vi "_DServerStart.vi"(3 "error in":errorcluster, 4 "instance name":string="unspecified_instance_name", 5 "executable name":string="unspecified_application_name") -> (0 "error out":errorcluster, 1 "device_list":string[](array[string]), 2 "dserver evt.":T1)   [LabVIEW 2014, in "tango.lvlib"]
uses:
  tango.lvlib
  Client Request Handling/Typedefs/_DServerEvent.ctl
  Client Request Handling/Typedefs/_DServerClientRequest.ctl
  Client Request Handling/Typedefs/_DServerClientRequestType.ctl
  Client Request Handling/Typedefs/_DServerClientRequestData.ctl
  Client Request Handling/Typedefs/_GenericDataBuffer.ctl
  Common VIs/Typedefs/_AttributeDataType_t.ctl
  tango_binding.so
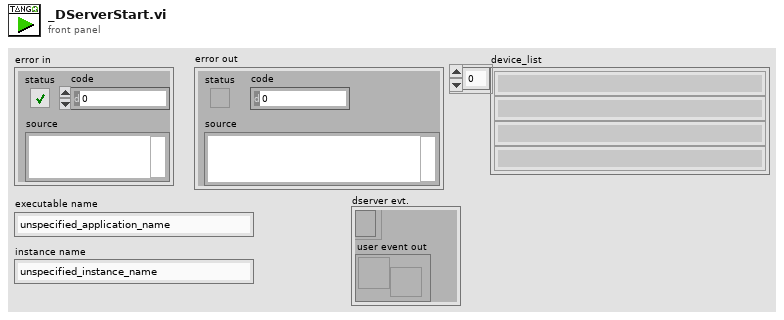
[diagram p1: front panel]
types:
  T1 = typedef "tango.lvlib/_DServerEvent.ctl" = cluster{"event registration refnum":refnum<event-registration>, "user event out":refnum<user-event>}
  T2 = cluster{"event registration refnum":refnum<event-registration>, "user event out":refnum<user-event>}
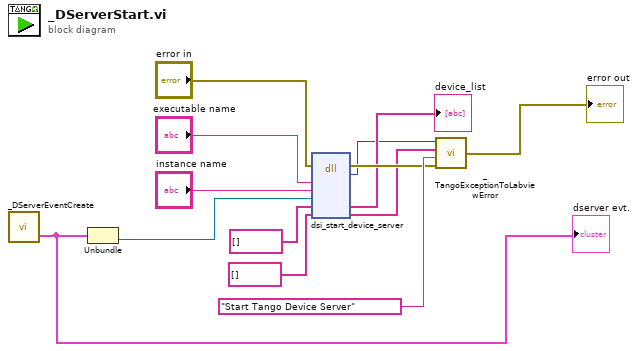
[diagram p0: block diagram]
diagram:
  n1 = call "_DServerEventCreate.vi"() -> ("dserver evt."=w1:T2)  [unwired: 1 in, 1 out]
  "dserver evt." <- w1
  n2 = Unbundle(w1) -> ("user event out"=w2:refnum<user-event>)  [unwired: 1 out]
  n3 = dll-call lib="tango_binding.*" fn="dsi_start_device_server"(error in="error in", "executable_name"="executable name", "instance_name"="instance name", "devicer_server_evt_ref"=w2, "device_list"=string[] [] ("error stack"), "error_stack"=string[] [] ("error stack")) -> (error out=w11:errorcluster, "return type"=w5:i32, "device_list"=→"device_list":string[], "error_stack"=w4:string[])  [unwired: 5 in, 1 out]
  n4 = call "_TangoExceptionToLabviewError.vi"("error in"=w11, "location"="Start Tango Device Server", "error stack"=w4, "error code"=w5) -> ("error out"=→"error out":errorcluster)
